vi "Does Wire Carry Typedef Data.vi"(6 "error in (no error)":errorcluster, 9 "Wire in":refnum<vi>) -> (0 "error out":errorcluster, 2 "Type":T1, 3 "Wire out":refnum<vi>, 4 "Type Definition/Class Path":string, 5 "Wire carry Typedef/Class":bool)   [LabVIEW 2020]
uses:
  <vilib>/Utility/Data Type/NI_Data Type.lvlib
  <vilib>/Utility/Data Type/Type Definitions/Data Type.ctl
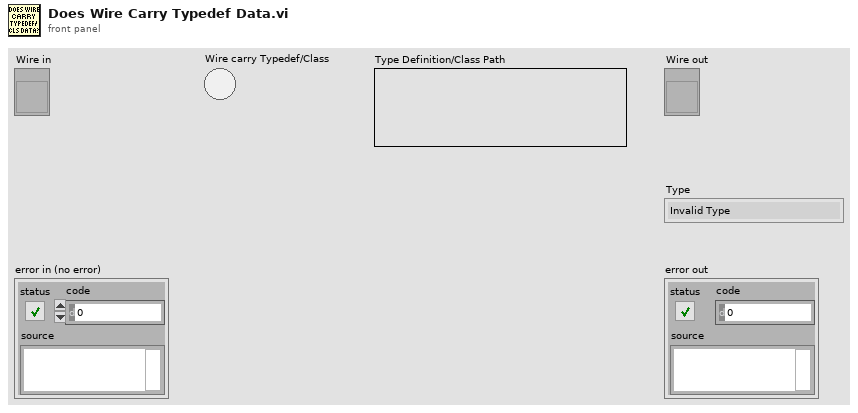
[diagram p1: front panel]
types:
  T1 = typedef "NI_Data Type.lvlib/Data Type.ctl" = enum8{"Invalid Type", "Void", "I8", "I16", "I32", "I64", "U8", "U16", "U32", "U64", "Single Float", "Double Float", "Extended Float", "Single Complex", "Double Complex", "Extended Complex", "Enum U8", "Enum U16", "Enum U32", "Enum U64", "Single Float With Unit", "Double Float With Unit", "Extended Float With Unit", "Single Complex with Unit", "Double Complex with Unit", "Extended Complex with Unit", "Boolean", "String", "Path", "Picture", "Tag", "Array", "Cluster", "Variant", "LV Variant", "Waveform", "Timestamp", "Digital Waveform", "Digital Data", "ExpressData", "Refnum", "External Data", "VI", "Poly VI", "LabVIEW Class Instance", "Fixed Point", "Set Collection", "Map Collection"}
  T2 = typedef "NI_Data Type.lvlib/Type Definition Info.ctl" = cluster{"Name":string, "Timestamp":u32}
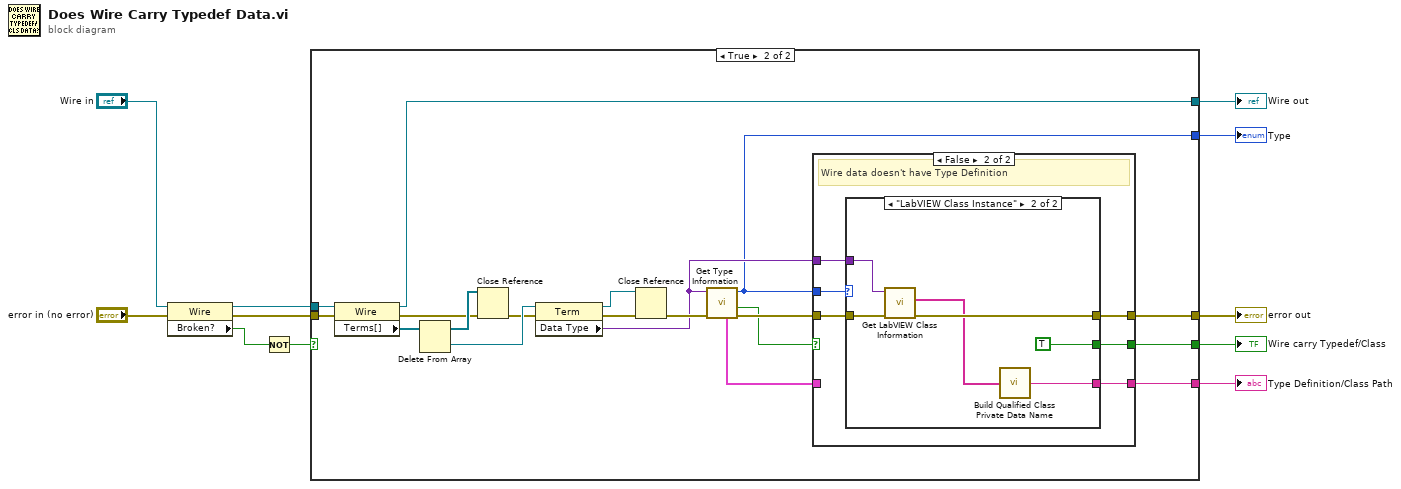
[diagram p0: block diagram]
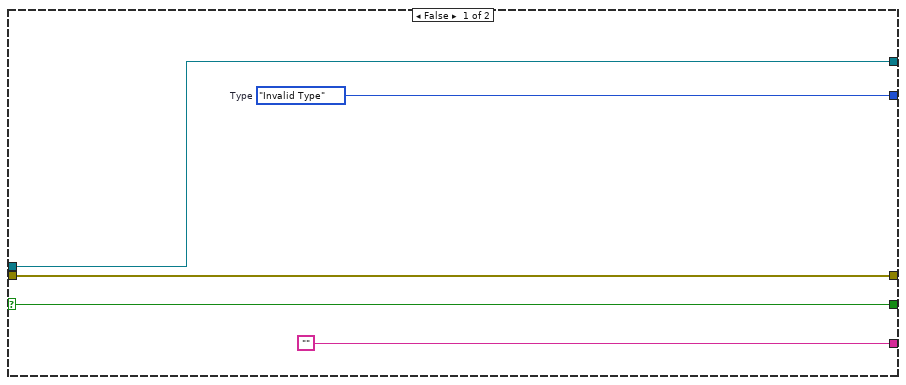
[diagram p2: hidden frame]
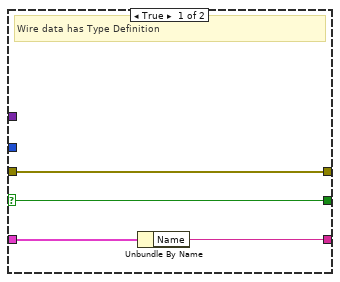
[diagram p3: hidden frame]
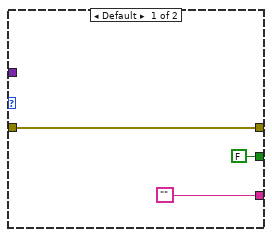
[diagram p4: hidden frame]
diagram:
  n1 = property class="Wire"(reference="Wire in", error in="error in (no error)") -> (reference out=w6:refnum<vi>, error out=w5:errorcluster, "Broken?"=w4:bool)
  n2 = Not(x=w4) -> (.not. x?=w7:bool)
  n3 = case shown="True" w7 {
    selector: w7 -> [w16 _]
    tunnel: w5 -> [w14 w35]
    tunnel: w6 -> [w15 w34]
    tunnel: [w16 w17] -> w8
    tunnel: [w15 w27] -> w9
    tunnel: [w14 w21] -> w10
    tunnel: ["" w23] -> w2
    tunnel: [w13 w18] -> w1
    frame False {
      w13 = Data_Type."Invalid Type"  # Type
    }
    frame True {
      n4 = property class="Wire"(reference=w34, error in=w35) -> (reference out=w27:refnum<vi>, error out=w31:errorcluster, "Terms[]"=w33:refnum<vi>[])
      n5 = Delete From Array(array=w33) -> (deleted portion=w30:refnum<vi>, array with subset deleted=w32:refnum<vi>[])  [unwired: 2 in]
      n6 = Close Reference(reference=w32, error in (no error)=w31) -> (error out=w29:errorcluster)
      n7 = property class="Term"(reference=w30, error in=w29) -> (reference out=w26:refnum<vi>, error out=w28:errorcluster, "Data Type"=w20:variant)
      n8 = Close Reference(reference=w26, error in (no error)=w28) -> (error out=w25:errorcluster)
      n9 = call <vilib>:"Get Type Information.vi"("error in (no error)"=w25, "variant"=w20) -> ("error out"=w22:errorcluster, "type definition"=w19:bool, "type"=w18:T1, "type definition info"=w24:T2)  [unwired: 5 in, 1 out]
      n10 = case shown="False" w19 {
        selector: w19 -> [w36 _]
        tunnel: w24 -> [w39 _]
        tunnel: [w38 w41] -> w23
        tunnel: w22 -> [w37 w45]
        tunnel: [w37 w44] -> w21
        tunnel: w20 -> [_ w43]
        tunnel: w18 -> [_ w42]
        tunnel: [w36 w40] -> w17
        frame True {
          # "Wire data has Type Definition"
          n11 = Unbundle By Name(w39) -> ("Name"=w38:string)
        }
        frame False {
          # "Wire data doesn't have Type Definition"
          n12 = case shown="\"LabVIEW Class Instance\"" w42 {
            tunnel: w45 -> [w48 w54]
            tunnel: [w48 w51] -> w44
            tunnel: w43 -> [_ w53]
            tunnel: ["" w49] -> w41
            tunnel: [FALSE TRUE] -> w40
            frame Default {
            }
            frame "LabVIEW Class Instance" {
              n13 = call <vilib>:"Get LabVIEW Class Information.vi"("error in (no error)"=w54, "variant"=w53) -> ("error out"=w51:errorcluster, "qualified LabVIEW class name"=w50:string[])  [unwired: 7 in, 1 out]
              n14 = call "Build Qualified Class Private Data Name.vi"("Qualified LabVIEW Class Name"=w50) -> ("Qualified LabVIEW Class Private Data Name"=w49:string)
            }
          }
        }
      }
    }
  }
  "error out" <- w10
  "Wire out" <- w9
  "Wire carry Typedef/Class" <- w8
  "Type Definition/Class Path" <- w2
  "Type" <- w1
